vi "Eric's Project Greedy Snake.vi"() -> ()   [LabVIEW 2020]
uses:
  <vilib>/event_ctls.llb/eventvkey.ctl
panel:
  out "String":string
  out "direction stored":enum16{"left", "right", "up", "down"}(ring)=enum."right"
  in  "stop game":bool
  in  "stop":bool
  in  "food?":bool=TRUE
  out "food location":i8[](array[numeric])
  out "snake coordinates":i8[][](array[numeric])
  out "VKey":T1
  in  "start":bool
  in  "Difficulty":enum16{"low", "midium", "high"}(ring)=enum."high"
  in  "direction":enum16{"left", "right", "up", "down"}(ring)=enum."right"
  in  "Boundary Height":i8=15 min=5 max=15
  in  "Boundary Width":i8=15 min=5 max=15
  out "map":bool[][](array[boolean])=[[FALSE, FALSE, FALSE, FALSE, FALSE, FALSE, FALSE, FALSE, FALSE, FALSE, FALSE, FALSE, FALSE, FALSE, FALSE], [FALSE, FALSE, FALSE, FALSE, FALSE, FALSE, FALSE, FALSE, FALSE, FALSE, FALSE, FALSE, FALSE, FALSE, FALSE], [FALSE, FALSE, FALSE, FALSE, FALSE, FALSE, FALSE, FALSE, FALSE, FALSE, FALSE, FALSE, FALSE, FALSE, FALSE], [FALSE, FALSE, FALSE, FALSE, FALSE, FALSE, FALSE, FALSE, FALSE, FALSE, FALSE, FALSE, FALSE, FALSE, FALSE], [FALSE, FALSE, FALSE, FALSE, FALSE, FALSE, FALSE, FALSE, FALSE, FALSE, FALSE, FALSE, FALSE, FALSE, FALSE], [FALSE, FALSE, FALSE, FALSE, FALSE, FALSE, FALSE, FALSE, FALSE, FALSE, FALSE, FALSE, FALSE, FALSE, FALSE], [FALSE, FALSE, FALSE, FALSE, FALSE, FALSE, FALSE, FALSE, FALSE, FALSE, FALSE, FALSE, FALSE, FALSE, FALSE], [FALSE, FALSE, FALSE, FALSE, FALSE, FALSE, TRUE, TRUE, FALSE, FALSE, FALSE, FALSE, FALSE, FALSE, FALSE], [FALSE, FALSE, FALSE, FALSE, FALSE, FALSE, FALSE, FALSE, FALSE, FALSE, FALSE, FALSE, FALSE, FALSE, FALSE], [FALSE, FALSE, FALSE, FALSE, FALSE, FALSE, FALSE, FALSE, FALSE, FALSE, FALSE, FALSE, FALSE, FALSE, FALSE], [FALSE, FALSE, FALSE, FALSE, FALSE, FALSE, FALSE, FALSE, FALSE, FALSE, FALSE, FALSE, FALSE, FALSE, FALSE], [FALSE, FALSE, FALSE, FALSE, FALSE, FALSE, FALSE, FALSE, FALSE, FALSE, FALSE, FALSE, FALSE, FALSE, FALSE], [FALSE, FALSE, FALSE, FALSE, FALSE, FALSE, FALSE, FALSE, FALSE, FALSE, FALSE, FALSE, FALSE, FALSE, FALSE], [FALSE, FALSE, FALSE, FALSE, FALSE, FALSE, FALSE, FALSE, FALSE, FALSE, FALSE, FALSE, FALSE, FALSE, FALSE], [FALSE, FALSE, FALSE, FALSE, FALSE, FALSE, FALSE, FALSE, FALSE, FALSE, FALSE, FALSE, FALSE, FALSE, FALSE]]
  # "maximun 15*15"
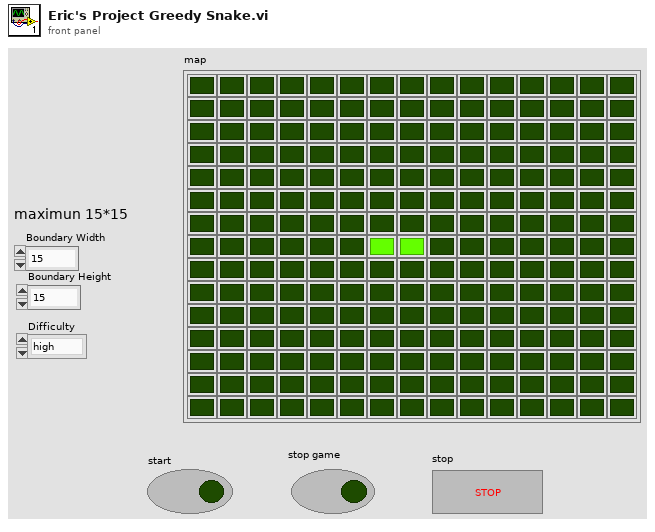
[diagram p1: front panel]
types:
  T1 = typedef "eventvkey.ctl" = enum16{"ASCII", "Enter", "Return", "Shift", "Ctrl", "Alt", "Cmd", "Opt", "Caps", "NumLock", "Clear", "Break", "Up", "Down", "Left", "Right", "Insert", "Delete", "Home", "End", "PageUp", "PageDown", "Escape", "Help", "Pause", "ScrollLock", "F1", "F2", "F3", "F4", "F5", "F6", "F7", "F8", "F9", "F10", "F11", "F12", "F13", "F14", "F15", "F16", "F17", "F18", "F19", "F20", "F21", "F22", "F23", "F24", "Play", "VolumeUp", "VolumeDown", "Mute", "Two Byte Char"}
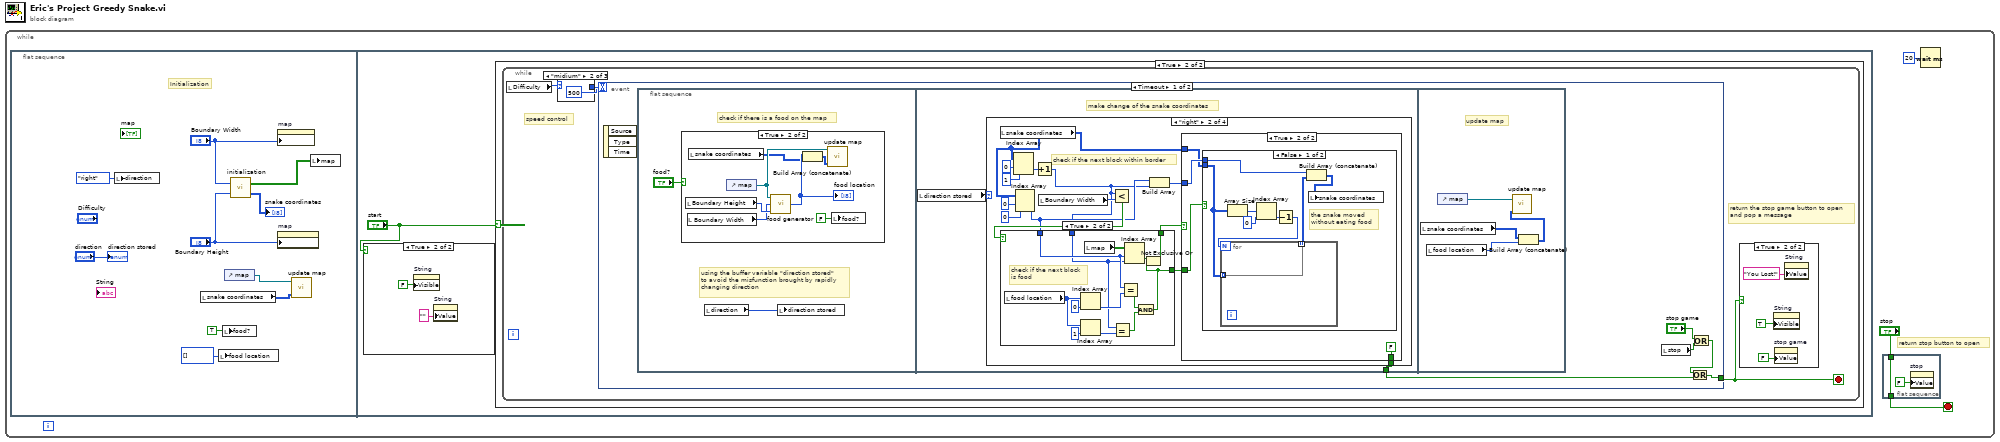
[diagram p0: block diagram]
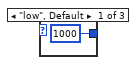
[diagram p5: hidden frame]
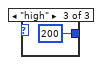
[diagram p6: hidden frame]
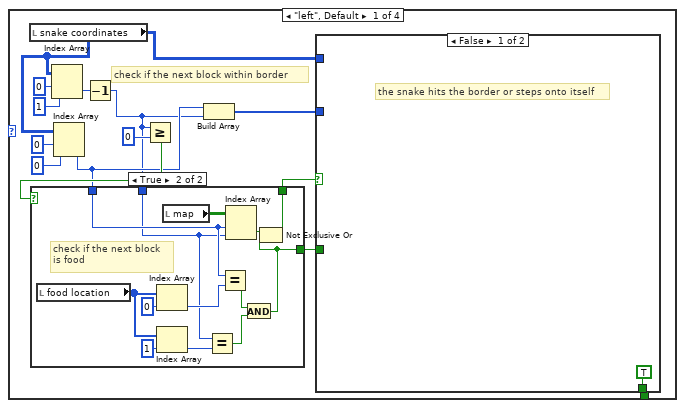
[diagram p8: hidden frame]
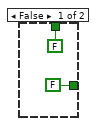
[diagram p9: hidden frame]
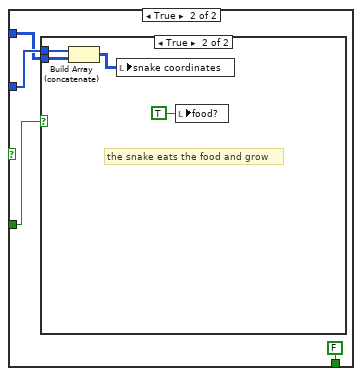
[diagram p10: hidden frame]
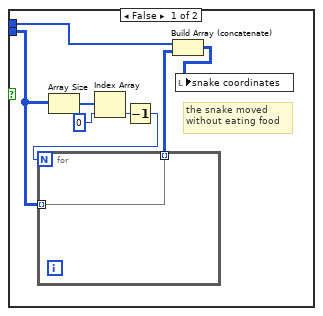
[diagram p11: hidden frame]
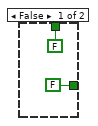
[diagram p12: hidden frame]
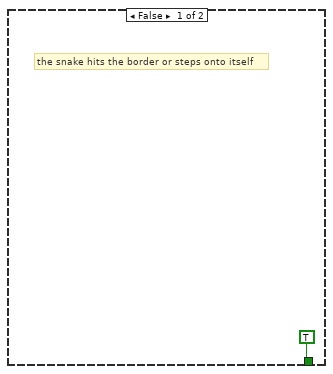
[diagram p13: hidden frame]
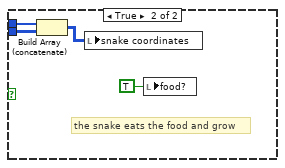
[diagram p14: hidden frame]
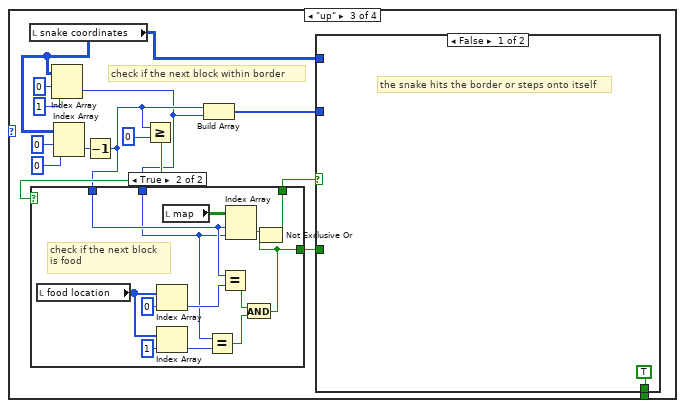
[diagram p15: hidden frame]
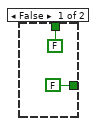
[diagram p16: hidden frame]
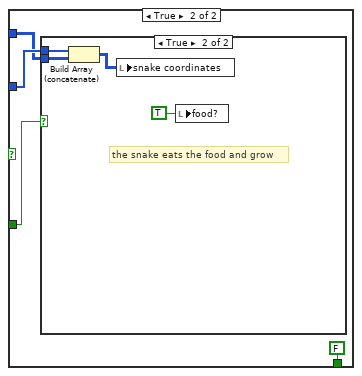
[diagram p17: hidden frame]
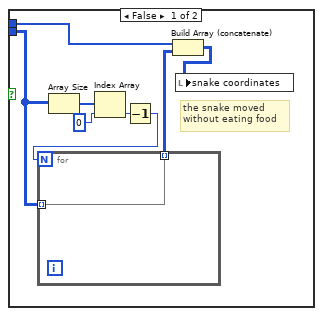
[diagram p18: hidden frame]
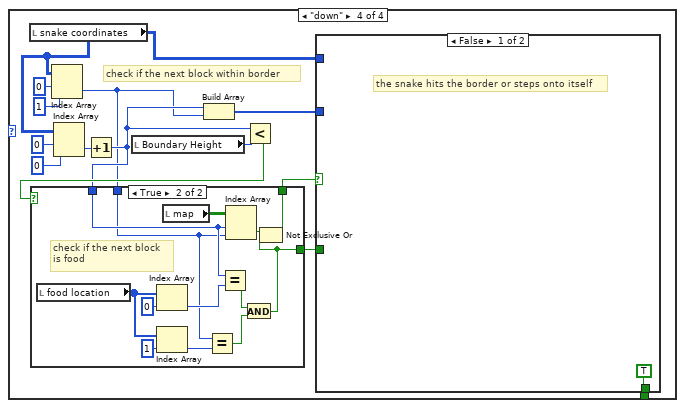
[diagram p19: hidden frame]
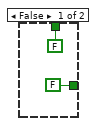
[diagram p20: hidden frame]
diagram:
  n1 = while {
    stop <- w2 stop-if-true
    # "return stop button to open"
    n2 = flat-sequence {
      frame #0 {
        # "Initialization"
        n3 = local write "direction"(enum16{"left", "right", "up", "down"}."right" ("direction")) -> ()
        n4 = local read "snake coordinates"() -> (w7:i8[][])
        n5 = local write "food location"(i8[] [] ("food location")) -> ()
        n6 = local write "food?"(TRUE ("food?")) -> ()
        n7 = control-ref of="map"() -> (w8:refnum<vi>)
        n8 = call "initialization.vi"("Boundary Height"="Boundary Height", "Boundary Width"="Boundary Width") -> ("snake coordinates"=→"snake coordinates":i8[][], "map"=w12:bool[][])
        n9 = property on="map" class="Arr (strict)"("Number of Columns"="Boundary Width") -> ()  [unwired: 2 in, 2 out]
        n10 = property on="map" class="Arr (strict)"("Number of Rows"="Boundary Height") -> ()  [unwired: 2 in, 2 out]
        n11 = call "update map.vi"("coordinates"=w7, "Array in"=w8) -> ()  [unwired: 1 in]
        n12 = local write "map"(w12) -> ()
        "direction stored" <- "direction"
      }
      frame #1 {
        n13 = case shown="True" "start" {
          frame False {
            # "change the user interface\n(no functional use right now)"
          }
          frame True {
            n14 = property on="String" class="Str"("Visible"=FALSE) -> ()  [unwired: 2 in, 2 out]
            n15 = property on="String" class="Str"("Value"="" ("String")) -> ()  [unwired: 2 in, 2 out]
          }
        }
        n16 = case shown="True" "start" {
          frame False {
          }
          frame True {
            n17 = while {
              stop <- w19 stop-if-true
              # "return the stop game button to open\nand pop a message"
              # "speed control"
              n18 = local read "Difficulty"() -> (w21:enum16{"low", "midium", "high"})
              n19 = case shown="\"midium\"" w21 {
                tunnel: [u32 1000 ("milliseconds to wait") u32 500 ("milliseconds to wait") u32 200 ("milliseconds to wait")] -> w20
                frame "low", Default {
                }
                frame "midium" {
                }
                frame "high" {
                }
              }
              n20 = event shown="[0] Timeout" {
                selector: _ -> [_ _]
                dyn-events: _ -> [_ _]
                timeout: w20 -> [_ _]
                tunnel: [w31 FALSE] -> w19
                event Timeout {
                  n21 = event-data() -> ()  [unwired: 1 in, 3 out]
                  n22 = flat-sequence {
                    tunnel: [w43] -> w32
                    frame #0 {
                      # "using the buffer variable \"direction stored\"\nto avoid the misfunction brought by rapidly\nchanging direction"
                      # "check if there is a food on the map"
                      n23 = case shown="True" "food?" {
                        frame False {
                        }
                        frame True {
                          n24 = local read "Boundary Height"() -> (w41:i8)
                          n25 = local read "Boundary Width"() -> (w40:i8)
                          n26 = local read "snake coordinates"() -> (w35:i8[][])
                          n27 = control-ref of="map"() -> (w37:refnum<vi>)
                          n28 = call "food generator.vi"("Boundary Height"=w41, "Boundary Width"=w40, "Array in"=w37) -> ("food location"=w39:i8[])
                          "food location" <- w39
                          n29 = Build Array (concatenate)(w39, w35) -> (w38:i8[][])
                          n30 = call "update map.vi"("coordinates"=w38, "Array in"=w37) -> ()  [unwired: 1 in]
                          n31 = local write "food?"(FALSE ("food?")) -> ()
                        }
                      }
                      n32 = local read "direction"() -> (w33:enum16{"left", "right", "up", "down"})
                      n33 = local write "direction stored"(w33) -> ()
                    }
                    frame #1 {
                      # "make change of the snake coordinates"
                      n34 = local read "direction stored"() -> (w42:enum16{"left", "right", "up", "down"})
                      n35 = case shown="\"right\"" w42 {
                        tunnel: [w48 w96 w143 w191] -> w43
                        frame "left", Default {
                          # "check if the next block within border"
                          n36 = local read "snake coordinates"() -> (w47:i8[][])
                          n37 = Index Array(array=w47, index (row)=0, index (col)=1 ("disabled index (col)")) -> (element=w55:i8)
                          n38 = Index Array(array=w47, index (row)=0, index (col)=0 ("disabled index (col)")) -> (element=w46:i8)
                          n39 = Decrement(x=w55) -> (x-1=w45:i8)
                          n40 = Greater Or Equal?(x=w45, y=i8 0) -> (x >= y?=w50:bool)
                          n41 = case shown="True" w50 {
                            tunnel: [FALSE w61] -> w49
                            tunnel: w46 -> [_ w69]
                            tunnel: w45 -> [_ w65]
                            tunnel: [FALSE w60] -> w52
                            frame False {
                            }
                            frame True {
                              # "check if the next block\nis food"
                              n42 = local read "food location"() -> (w67:i8[])
                              n43 = Index Array(array=w67, index=0) -> (element=w70:i8)
                              n44 = Index Array(array=w67, index=1) -> (element=w66:i8)
                              n45 = local read "map"() -> (w72:bool[][])
                              n46 = Equal?(x=w65, y=w66) -> (x = y?=w63:bool)
                              n47 = Equal?(x=w69, y=w70) -> (x = y?=w64:bool)
                              n48 = Index Array(array=w72, index (row)=w69, index (col)=w65) -> (element=w62:bool)
                              n49 = And(x=w64, y=w63) -> (x .and. y?=w60:bool)
                              n50 = Not Exclusive Or(1:w60, 2:w62) -> (0:w61:bool)
                            }
                          }
                          n51 = Build Array(w46, w45) -> (w44:i8[])
                          n52 = case shown="False" w49 {
                            tunnel: w52 -> [_ w74]
                            tunnel: [TRUE FALSE] -> w48
                            tunnel: w47 -> [_ w75]
                            tunnel: w44 -> [_ w76]
                            frame False {
                              # "the snake hits the border or steps onto itself"
                            }
                            frame True {
                              n53 = case shown="True" w74 {
                                tunnel: w76 -> [w80 w90]
                                tunnel: w75 -> [w85 w89]
                                frame False {
                                # "the snake moved \nwithout eating food"
                                n54 = Array Size(array=w85) -> (size(s)=w84:i32[])
                                n55 = Index Array(array=w84, index=0) -> (element=w82:i32)
                                n56 = Decrement(x=w82) -> (x-1=w81:i32)
                                n57 = for {
                                N: w81 -> [_]
                                tunnel: w85 -> [w86] mode=indexing
                                tunnel: [w86] -> w79 mode=indexing
                                }
                                n58 = Build Array (concatenate)(w80, w79) -> (w78:i8[][])
                                n59 = local write "snake coordinates"(w78) -> ()
                                }
                                frame True {
                                # "the snake eats the food and grow"
                                n60 = Build Array (concatenate)(w90, w89) -> (w87:i8[][])
                                n61 = local write "snake coordinates"(w87) -> ()
                                n62 = local write "food?"(TRUE ("food?")) -> ()
                                }
                              }
                            }
                          }
                        }
                        frame "right" {
                          # "check if the next block within border"
                          n63 = local read "snake coordinates"() -> (w95:i8[][])
                          n64 = Index Array(array=w95, index (row)=0, index (col)=1 ("disabled index (col)")) -> (element=w102:i8)
                          n65 = Index Array(array=w95, index (row)=0, index (col)=0 ("disabled index (col)")) -> (element=w94:i8)
                          n66 = Increment(x=w102) -> (x+1=w91:i8)
                          n67 = local read "Boundary Width"() -> (w92:i8)
                          n68 = Less?(x=w91, y=w92) -> (x < y?=w98:bool)
                          n69 = case shown="True" w98 {
                            tunnel: [FALSE w108] -> w97
                            tunnel: w94 -> [_ w116]
                            tunnel: w91 -> [_ w112]
                            tunnel: [FALSE w107] -> w99
                            frame False {
                            }
                            frame True {
                              # "check if the next block\nis food"
                              n70 = local read "food location"() -> (w114:i8[])
                              n71 = Index Array(array=w114, index=0) -> (element=w117:i8)
                              n72 = Index Array(array=w114, index=1) -> (element=w113:i8)
                              n73 = local read "map"() -> (w119:bool[][])
                              n74 = Equal?(x=w112, y=w113) -> (x = y?=w110:bool)
                              n75 = Equal?(x=w116, y=w117) -> (x = y?=w111:bool)
                              n76 = Index Array(array=w119, index (row)=w116, index (col)=w112) -> (element=w109:bool)
                              n77 = And(x=w111, y=w110) -> (x .and. y?=w107:bool)
                              n78 = Not Exclusive Or(1:w107, 2:w109) -> (0:w108:bool)
                            }
                          }
                          n79 = Build Array(w94, w91) -> (w93:i8[])
                          n80 = case shown="True" w97 {
                            tunnel: w99 -> [_ w122]
                            tunnel: [TRUE FALSE] -> w96
                            tunnel: w95 -> [_ w123]
                            tunnel: w93 -> [_ w124]
                            frame False {
                              # "the snake hits the border or steps onto itself"
                            }
                            frame True {
                              n81 = case shown="False" w122 {
                                tunnel: w124 -> [w127 w137]
                                tunnel: w123 -> [w132 w136]
                                frame False {
                                # "the snake moved \nwithout eating food"
                                n82 = Array Size(array=w132) -> (size(s)=w131:i32[])
                                n83 = Index Array(array=w131, index=0) -> (element=w129:i32)
                                n84 = Decrement(x=w129) -> (x-1=w128:i32)
                                n85 = for {
                                N: w128 -> [_]
                                tunnel: w132 -> [w133] mode=indexing
                                tunnel: [w133] -> w126 mode=indexing
                                }
                                n86 = Build Array (concatenate)(w127, w126) -> (w125:i8[][])
                                n87 = local write "snake coordinates"(w125) -> ()
                                }
                                frame True {
                                # "the snake eats the food and grow"
                                n88 = Build Array (concatenate)(w137, w136) -> (w134:i8[][])
                                n89 = local write "snake coordinates"(w134) -> ()
                                n90 = local write "food?"(TRUE ("food?")) -> ()
                                }
                              }
                            }
                          }
                        }
                        frame "up" {
                          # "check if the next block within border"
                          n91 = local read "snake coordinates"() -> (w142:i8[][])
                          n92 = Index Array(array=w142, index (row)=0, index (col)=1 ("disabled index (col)")) -> (element=w138:i8)
                          n93 = Index Array(array=w142, index (row)=0, index (col)=0 ("disabled index (col)")) -> (element=w140:i8)
                          n94 = Decrement(x=w140) -> (x-1=w139:i8)
                          n95 = Greater Or Equal?(x=w139, y=i8 0) -> (x >= y?=w145:bool)
                          n96 = case shown="True" w145 {
                            tunnel: [FALSE w155] -> w144
                            tunnel: w139 -> [_ w163]
                            tunnel: w138 -> [_ w159]
                            tunnel: [FALSE w154] -> w147
                            frame False {
                            }
                            frame True {
                              # "check if the next block\nis food"
                              n97 = local read "food location"() -> (w161:i8[])
                              n98 = Index Array(array=w161, index=0) -> (element=w164:i8)
                              n99 = Index Array(array=w161, index=1) -> (element=w160:i8)
                              n100 = local read "map"() -> (w166:bool[][])
                              n101 = Equal?(x=w159, y=w160) -> (x = y?=w157:bool)
                              n102 = Equal?(x=w163, y=w164) -> (x = y?=w158:bool)
                              n103 = Index Array(array=w166, index (row)=w163, index (col)=w159) -> (element=w156:bool)
                              n104 = And(x=w158, y=w157) -> (x .and. y?=w154:bool)
                              n105 = Not Exclusive Or(1:w154, 2:w156) -> (0:w155:bool)
                            }
                          }
                          n106 = Build Array(w139, w138) -> (w141:i8[])
                          n107 = case shown="False" w144 {
                            tunnel: w147 -> [_ w168]
                            tunnel: [TRUE FALSE] -> w143
                            tunnel: w142 -> [_ w169]
                            tunnel: w141 -> [_ w170]
                            frame False {
                              # "the snake hits the border or steps onto itself"
                            }
                            frame True {
                              n108 = case shown="True" w168 {
                                tunnel: w170 -> [w174 w184]
                                tunnel: w169 -> [w179 w183]
                                frame False {
                                # "the snake moved \nwithout eating food"
                                n109 = Array Size(array=w179) -> (size(s)=w178:i32[])
                                n110 = Index Array(array=w178, index=0) -> (element=w176:i32)
                                n111 = Decrement(x=w176) -> (x-1=w175:i32)
                                n112 = for {
                                N: w175 -> [_]
                                tunnel: w179 -> [w180] mode=indexing
                                tunnel: [w180] -> w173 mode=indexing
                                }
                                n113 = Build Array (concatenate)(w174, w173) -> (w172:i8[][])
                                n114 = local write "snake coordinates"(w172) -> ()
                                }
                                frame True {
                                # "the snake eats the food and grow"
                                n115 = Build Array (concatenate)(w184, w183) -> (w181:i8[][])
                                n116 = local write "snake coordinates"(w181) -> ()
                                n117 = local write "food?"(TRUE ("food?")) -> ()
                                }
                              }
                            }
                          }
                        }
                        frame "down" {
                          # "check if the next block within border"
                          n118 = local read "snake coordinates"() -> (w190:i8[][])
                          n119 = Index Array(array=w190, index (row)=0, index (col)=1 ("disabled index (col)")) -> (element=w185:i8)
                          n120 = Index Array(array=w190, index (row)=0, index (col)=0 ("disabled index (col)")) -> (element=w188:i8)
                          n121 = Increment(x=w188) -> (x+1=w186:i8)
                          n122 = local read "Boundary Height"() -> (w187:i8)
                          n123 = Build Array(w186, w185) -> (w189:i8[])
                          n124 = Less?(x=w186, y=w187) -> (x < y?=w193:bool)
                          n125 = case shown="True" w193 {
                            tunnel: [FALSE w202] -> w192
                            tunnel: w186 -> [_ w210]
                            tunnel: w185 -> [_ w206]
                            tunnel: [FALSE w201] -> w194
                            frame False {
                            }
                            frame True {
                              # "check if the next block\nis food"
                              n126 = local read "food location"() -> (w208:i8[])
                              n127 = Index Array(array=w208, index=0) -> (element=w211:i8)
                              n128 = Index Array(array=w208, index=1) -> (element=w207:i8)
                              n129 = local read "map"() -> (w213:bool[][])
                              n130 = Equal?(x=w206, y=w207) -> (x = y?=w204:bool)
                              n131 = Equal?(x=w210, y=w211) -> (x = y?=w205:bool)
                              n132 = Index Array(array=w213, index (row)=w210, index (col)=w206) -> (element=w203:bool)
                              n133 = And(x=w205, y=w204) -> (x .and. y?=w201:bool)
                              n134 = Not Exclusive Or(1:w201, 2:w203) -> (0:w202:bool)
                            }
                          }
                          n135 = case shown="False" w192 {
                            tunnel: w194 -> [_ w215]
                            tunnel: [TRUE FALSE] -> w191
                            tunnel: w190 -> [_ w216]
                            tunnel: w189 -> [_ w217]
                            frame False {
                              # "the snake hits the border or steps onto itself"
                            }
                            frame True {
                              n136 = case shown="False" w215 {
                                tunnel: w217 -> [w221 w231]
                                tunnel: w216 -> [w226 w230]
                                frame False {
                                # "the snake moved \nwithout eating food"
                                n137 = Array Size(array=w226) -> (size(s)=w225:i32[])
                                n138 = Index Array(array=w225, index=0) -> (element=w223:i32)
                                n139 = Decrement(x=w223) -> (x-1=w222:i32)
                                n140 = for {
                                N: w222 -> [_]
                                tunnel: w226 -> [w227] mode=indexing
                                tunnel: [w227] -> w220 mode=indexing
                                }
                                n141 = Build Array (concatenate)(w221, w220) -> (w219:i8[][])
                                n142 = local write "snake coordinates"(w219) -> ()
                                }
                                frame True {
                                # "the snake eats the food and grow"
                                n143 = Build Array (concatenate)(w231, w230) -> (w228:i8[][])
                                n144 = local write "snake coordinates"(w228) -> ()
                                n145 = local write "food?"(TRUE ("food?")) -> ()
                                }
                              }
                            }
                          }
                        }
                      }
                    }
                    frame #2 {
                      # "update map"
                      n146 = local read "snake coordinates"() -> (w234:i8[][])
                      n147 = local read "food location"() -> (w235:i8[])
                      n148 = control-ref of="map"() -> (w233:refnum<vi>)
                      n149 = Build Array (concatenate)(w234, w235) -> (w232:i8[][])
                      n150 = call "update map.vi"("coordinates"=w232, "Array in"=w233) -> ()  [unwired: 1 in]
                    }
                  }
                  n151 = local read "stop"() -> (w30:bool)
                  n152 = Or(x="stop game", y=w30) -> (x .or. y?=w28:bool)
                  n153 = Or(x=w28, y=w32) -> (x .or. y?=w31:bool)
                }
                event Key Down {
                  # "the buffer variable prevents the user\nfrom changing to an illegal direction\nthat may end the game(say from left to right)"
                  # "change direction of the snakes movement"
                  n154 = event-data() -> ("VKey"=→"VKey":T1)  [unwired: 1 in, 9 out]
                  n155 = local read "direction stored"() -> (w236:enum16{"left", "right", "up", "down"})
                  n156 = local read "VKey"() -> (w238:T1)
                  n157 = case shown="\"right\"" w236 {
                    tunnel: w238 -> [w242 w247 w252 w257]
                    tunnel: [w241 w246 w251 w256] -> w240
                    frame "left", Default {
                      n158 = case shown="\"Up\"" w242 {
                        tunnel: [w243 enum16{"left", "right", "up", "down"}."up" ("direction") enum16{"left", "right", "up", "down"}."down" ("direction")] -> w241
                        frame "Insert", Default {
                          n159 = local read "direction"() -> (w243:enum16{"left", "right", "up", "down"})
                        }
                        frame "Up" {
                        }
                        frame "Down" {
                        }
                      }
                    }
                    frame "right" {
                      n160 = case shown="\"Up\"" w247 {
                        tunnel: [w248 enum16{"left", "right", "up", "down"}."up" ("direction") enum16{"left", "right", "up", "down"}."down" ("direction")] -> w246
                        frame "Insert", Default {
                          n161 = local read "direction"() -> (w248:enum16{"left", "right", "up", "down"})
                        }
                        frame "Up" {
                        }
                        frame "Down" {
                        }
                      }
                    }
                    frame "up" {
                      n162 = case shown="\"Right\"" w252 {
                        tunnel: [w253 enum16{"left", "right", "up", "down"}."left" ("direction") enum16{"left", "right", "up", "down"}."right" ("direction")] -> w251
                        frame "Insert", Default {
                          n163 = local read "direction"() -> (w253:enum16{"left", "right", "up", "down"})
                        }
                        frame "Left" {
                        }
                        frame "Right" {
                        }
                      }
                    }
                    frame "down" {
                      n164 = case shown="\"Left\"" w257 {
                        tunnel: [w258 enum16{"left", "right", "up", "down"}."left" ("direction") enum16{"left", "right", "up", "down"}."right" ("direction")] -> w256
                        frame "Insert", Default {
                          n165 = local read "direction"() -> (w258:enum16{"left", "right", "up", "down"})
                        }
                        frame "Left" {
                        }
                        frame "Right" {
                        }
                      }
                    }
                  }
                  n166 = local write "direction"(w240) -> ()
                }
              }
              n167 = case shown="True" w19 {
                frame False {
                }
                frame True {
                  n168 = property on="String" class="Str"("Visible"=TRUE) -> ()  [unwired: 2 in, 2 out]
                  n169 = property on="stop game" class="Bool (strict)"("Value"=FALSE ("stop game")) -> ()  [unwired: 2 in, 2 out]
                  n170 = property on="String" class="Str"("Value"="You Lost!" ("String")) -> ()  [unwired: 2 in, 2 out]
                }
              }
            }
          }
        }
      }
    }
    n171 = flat-sequence {
      tunnel: "stop" -> [w4]
      tunnel: [w4] -> w2
      frame #0 {
        n172 = property on="stop" class="Bool (strict)"("Value"=FALSE ("stop")) -> ()  [unwired: 2 in, 2 out]
      }
    }
    n173 = Wait (ms)(milliseconds to wait=u32 20) -> ()  [unwired: 1 out]
  }
